vi "Update Status_.vi"(8 "error in (no error)":errorcluster, 11 "DAQmxTaksContainer_General in":refnum<class "DAQmxTaksContainer_General.lvclass">) -> (0 "error out":errorcluster, 3 "DAQmxTaksContainer_General out":refnum<class "DAQmxTaksContainer_General.lvclass">)   [LabVIEW 2019, in "DAQmxTaksContainer_General.lvclass"]
uses:
  DAQmxTaksContainer_General.lvclass
  DAQmxTaksContainer_General.lvclass/DAQmxTaksContainer_General.ctl
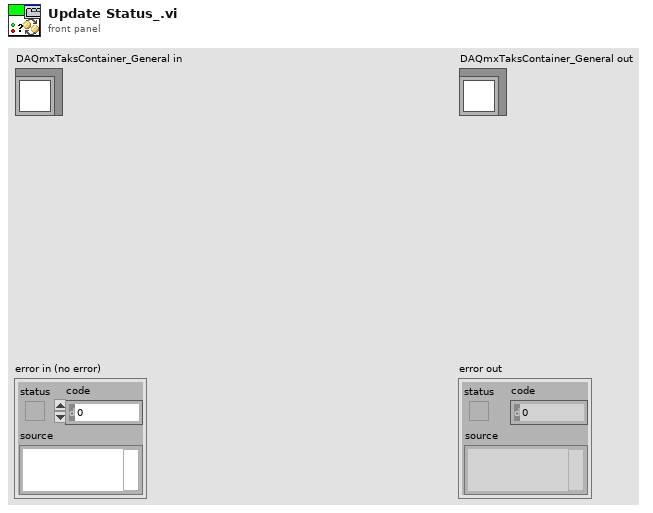
[diagram p1: front panel]
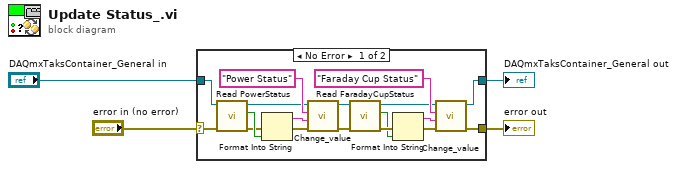
[diagram p0: block diagram]
diagram:
  n1 = case shown="No Error" "error in (no error)" {
    selector: "error in (no error)" -> [w20 w23]
    tunnel: [w14 w24] -> w2
    tunnel: "DAQmxTaksContainer_General in" -> [w21 w24]
    tunnel: [w15 w23] -> w1
    frame No Error {
      n2 = call "Read PowerStatus.vi"("error in (no error)"=w20, "DAQmxTaksContainer_General in"=w21) -> ("error out"=w11:errorcluster, "PowerStatus"=w22:bool, "DAQmxTaksContainer_General out"=w10:refnum<class "DAQmxTaksContainer_General.lvclass">)  [unwired: 7 in]
      n3 = Format Into String(error in=w11, w22) -> (resulting string=w18:string, error out=w13:errorcluster)  [unwired: 2 in]
      n4 = call-dynamic "Change_value.vi"("error in (no error)"=w13, "Data string"=w18, "Task name"="Power Status", "DAQmxTaksContainer_General in"=w10) -> ("error out"=w8:errorcluster, "DAQmxTaksContainer_General out"=w9:refnum<class "DAQmxTaksContainer_General.lvclass">)  [unwired: 6 in]
      n5 = call "Read FaradayCupStatus.vi"("error in (no error)"=w8, "DAQmxTaksContainer_General in"=w9) -> ("error out"=w7:errorcluster, "FaradayCupStatus"=w5:bool, "DAQmxTaksContainer_General out"=w6:refnum<class "DAQmxTaksContainer_General.lvclass">)  [unwired: 7 in]
      n6 = Format Into String(error in=w7, w5) -> (resulting string=w17:string, error out=w12:errorcluster)  [unwired: 2 in]
      n7 = call-dynamic "Change_value.vi"("error in (no error)"=w12, "Data string"=w17, "Task name"="Faraday Cup Status", "DAQmxTaksContainer_General in"=w6) -> ("error out"=w15:errorcluster, "DAQmxTaksContainer_General out"=w14:refnum<class "DAQmxTaksContainer_General.lvclass">)  [unwired: 6 in]
    }
    frame Error {
    }
  }
  "error out" <- w1
  "DAQmxTaksContainer_General out" <- w2
